vi "Untitled 1.vi"() -> ()   [LabVIEW 2021]
panel:
  out "Sync OK":bool
  out "Time After Sync":timestamp
  out "Time Before Sync":timestamp
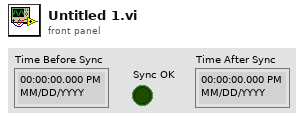
[diagram p1: front panel]
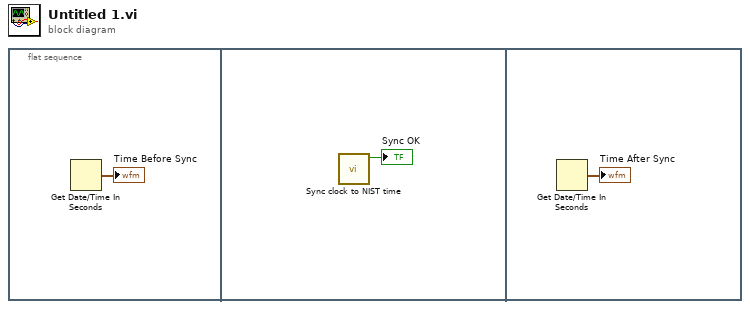
[diagram p0: block diagram]
diagram:
  n1 = flat-sequence {
    frame #0 {
      n2 = Get Date/Time In Seconds() -> (seconds since 1Jan1904=→"Time Before Sync":timestamp)
    }
    frame #1 {
      n3 = call "Sync clock to NIST time.vi"() -> ("Sync OK"=→"Sync OK":bool)  [unwired: 11 in]
    }
    frame #2 {
      n4 = Get Date/Time In Seconds() -> (seconds since 1Jan1904=→"Time After Sync":timestamp)
    }
  }
